vi "Set Horizontal Step Size.vi"(8 "error in":errorcluster, 10 "horizontal step size":i16, 11 "eye scan in":refnum<class "niHighSpeedSerial Rectangular Eye Scan v1 Host.lvclass">) -> (0 "error out":errorcluster, 3 "eye scan out":refnum<class "niHighSpeedSerial Rectangular Eye Scan v1 Host.lvclass">)   [LabVIEW 2014, in "niHighSpeedSerial Rectangular Eye Scan v1 Host.lvclass"]
doc: "Returns the horizontal step size.\n\n<B>Input Parameters</B>\n\n<B>eye scan in</B> Takes in a reference to your session from the previous VI.\n\n<B>error in</B> describes error conditions that occur before this node runs. This input provides standard 'error in' functionality.\n\n<B>horizontal step size</B> is the number of offsets to skip between each point on the horizontal axis.\n\n<B>Output Parameters</B>\n\n<B>eye scan out</B> passes a reference to your session to the next VI.\n\n<B>error out</B> contains error information. This output provides standard 'error out' functionality."
uses:
  <instrlib>/niHighSpeedSerial/Eye Scan/v1/Host/Impl/Rectangular Eye Scan/niHighSpeedSerial Rectangular Eye Scan v1 Host.lvclass
  <instrlib>/niHighSpeedSerial/Eye Scan/v1/Host/Impl/Rectangular Eye Scan/niHighSpeedSerial Rectangular Eye Scan v1 Host.lvclass/niHighSpeedSerial Rectangular Eye Scan v1 Host.ctl
  <vilib>/Utility/error.llb/Error Cluster From Error Code.vi
  <vilib>/ErrorRing/Error Ring.xnode
  <instrlib>/niHighSpeedSerial/Eye Scan/v1/Host/Eye Scan/niHighSpeedSerial Eye Scan v1 Host.lvclass
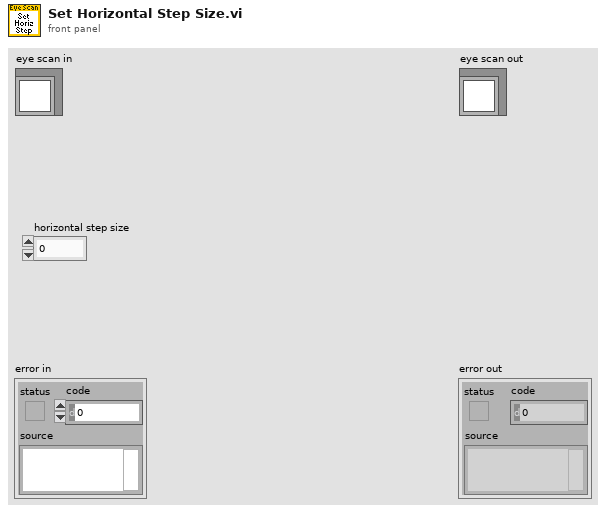
[diagram p1: front panel]
types:
  T1 = typedef "Rectangular Eye Scan v1 Host.lvclass/Private Data.ctl" = cluster{"horizontal step size":i16, "vertical step size":i16, "rectangular eye scan point iterator":refnum<class "niHighSpeedSerial Rectangular Eye Scan Point Iterator v1 Host.lvclass">}
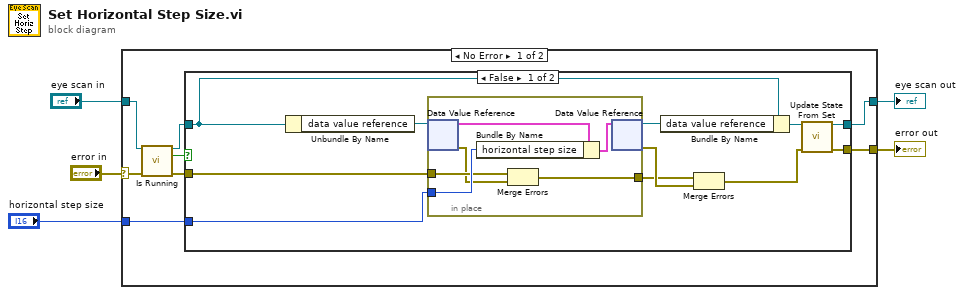
[diagram p0: block diagram]
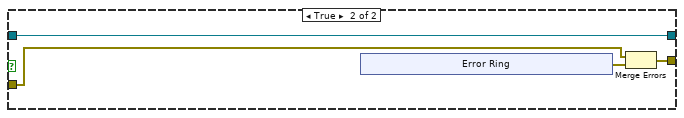
[diagram p2: hidden frame]
diagram:
  n1 = case shown="No Error" "error in" {
    selector: "error in" -> [w9 w40]
    tunnel: [w11 w40] -> w4
    tunnel: [w13 w39] -> w2
    tunnel: "eye scan in" -> [w10 w39]
    tunnel: "horizontal step size" -> [w12 _]
    frame No Error {
      n2 = call <instrlib>:"Is Running.vi"("eye scan in"=w10, "error in"=w9) -> ("eye scan out"=w7:refnum<class "niHighSpeedSerial Rectangular Eye Scan v1 Host.lvclass">, "is running?"=w6:bool, "error out"=w8:errorcluster)  [unwired: 11 in]
      n3 = case shown="False" w6 {
        tunnel: [w15 w33] -> w13
        tunnel: w7 -> [w22 w33]
        tunnel: w12 -> [w21 _]
        tunnel: w8 -> [w20 w34]
        tunnel: [w16 w32] -> w11
        frame False {
          n4 = Unbundle By Name(w22) -> ("data value reference"=w24:refnum<data-value>)
          n5 = in-place {
            in-place-border: w21 -> [w29]
            in-place-border: w20 -> [w27]
            in-place-border: [w25] -> w18
            n6 = in-place-dvr #1(w24) -> (w30:T1, w26:errorcluster)
            n7 = Bundle By Name(cluster=w30, "horizontal step size"=w29) -> (w28:T1)
            n8 = Merge Errors(w27, w26) -> (w25:errorcluster)
            n9 = in-place-dvr #1(w28) -> (w23:refnum<data-value>, w19:errorcluster)
          }
          n10 = Bundle By Name(cluster=w22, "data value reference"=w23) -> (w14:refnum<class "niHighSpeedSerial Rectangular Eye Scan v1 Host.lvclass">)
          n11 = Merge Errors(w18, w19) -> (w17:errorcluster)
          n12 = call <instrlib>:"Update State From Set.vi"("eye scan in"=w14, "error in"=w17) -> ("eye scan out"=w15:refnum<class "niHighSpeedSerial Rectangular Eye Scan v1 Host.lvclass">, "error out"=w16:errorcluster)  [unwired: 12 in]
        }
        frame True {
          n13 = xnode "Error Ring"() -> ("error out"=w31:errorcluster)
          n14 = Merge Errors(w34, w31) -> (w32:errorcluster)
        }
      }
    }
    frame Error {
    }
  }
  "error out" <- w4
  "eye scan out" <- w2
